vi "Bounded Confidence interval.vi"(1 "Analysis_info_cluster":T1={"Colour"=0, "Inst type"=enum."Pitot-static tube", "Inst name"="Manometer voltage", "Symbol"="U", "Code name"="", "Extra Info"="U", "Inst Array"=enum."PWA", "U"=0.0, "u^2"=0.0, "u^3"=0.0, "u^4"=0.0, "Skew_u"=0.0, "Kurt_u"=0.0, "Sd Error in Mean"=0.0, "% u'/U"=0.0, "X"=0.0, "Y"=0.0, "Z"=0.0, "Timescale integral Estimate"=0.0, "Sd Error in Variance"=0.0, "Calib File"=path "", "Calib Constants"=[], "Output Position"=FALSE, "Stats"=enum."None", "Av Sampling Rate"=0.0, "Av No of Samples"=0.0, "Total Meas Time (s)"=0.0, "OrigChName"="", "Max value"=0.0, "Min value"=0.0, "Req Sample Rate Hz"=0.0, "Sync Delay Time (s)"=0.0, "Ch No"=0, "Device"="", "Use Latest Calib"=FALSE, "Port"="", "Metadata Ch Names"=[], "Metadata Ch Values"=[], "Label"="", "chState"=enum."Solo", "Point Drift"=0.0, "inputConfig"=""} {"Kurt_u" format="%_3g"; "u^4" format="%_3g"; "u^3" format="%_3g"; "Sd Error in Variance" format="%_3g"; "u^2" format="%_3g"; "Sd Error in Mean" format="%_3g"; "U" format="%_3g"; "Sync Delay Time (s)" format="%.4f"; "Total Meas Time (s)" format="%_5g"; "Skew_u" format="%_3g"; "% u'/U" format="%_3g"}, 2 "Lower limit scale factor on SD or SE":dbl, 3 "Upper limit scale factor on SD or SE":dbl) -> (0 "Error values":string[](array[string]))   [LabVIEW 2022 SP3]
uses:
  Controls/Inst_type.ctl
  Controls/Instrument_Array.ctl
  Controls/Analysis_info_cluster.ctl
  Controls/channelState.ctl
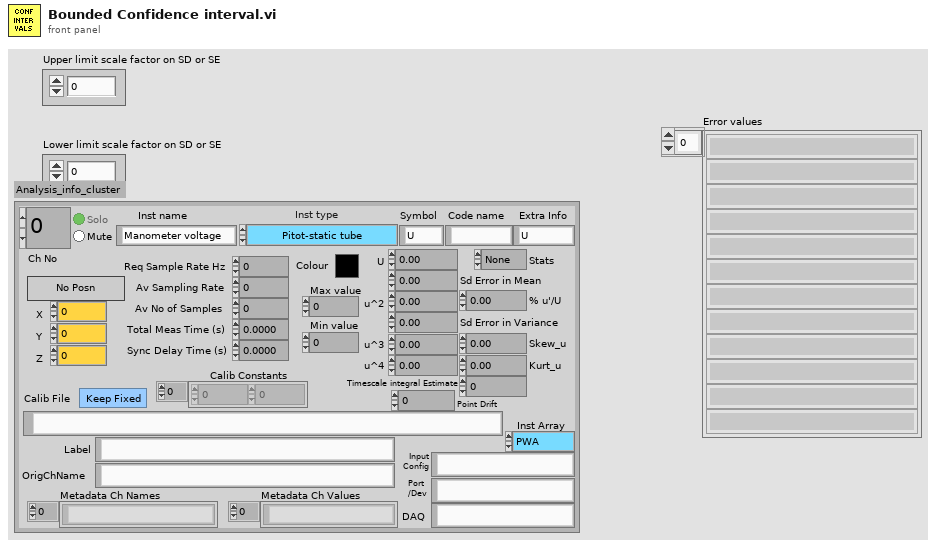
[diagram p1: front panel]
types:
  T1 = typedef "Analysis_info_cluster.ctl" = cluster{"Colour":u32, "Inst type":T2, "Inst name":string, "Symbol":string, "Code name":string, "Extra Info":string, "Inst Array":T3, "U":dbl, "u^2":dbl, "u^3":dbl, "u^4":dbl, "Skew_u":dbl, "Kurt_u":dbl, "Sd Error in Mean":dbl, "% u'/U":dbl, "X":dbl, "Y":dbl, "Z":dbl, "Timescale integral Estimate":dbl, "Sd Error in Variance":dbl, "Calib File":path, "Calib Constants":dbl[], "Output Position":bool, "Stats":enum16{"None", "Basic", "Full"}, "Av Sampling Rate":dbl, "Av No of Samples":dbl, "Total Meas Time (s)":dbl, "OrigChName":string, "Max value":dbl, "Min value":dbl, "Req Sample Rate Hz":dbl, "Sync Delay Time (s)":dbl, "Ch No":i16, "Device":string, "Use Latest Calib":bool, "Port":string, "Metadata Ch Names":string[], "Metadata Ch Values":string[], "Label":string, "chState":T4, "Point Drift":dbl, "inputConfig":string}
  T2 = typedef "Inst_type.ctl" = enum16{"Raw voltage", "Raw with zero offsetting", "Propeller anemometer", "Pressure Transducer", "Pitot-static tube", "Hot wire", "Cross wire 1", "Cross wire 2", "Generic Linear", "Generic Polynomial", "Generic BackPoly", "Fast FID", "Thermocouple", "Cold wire", "Pulsed Wire", "LDA Vel", "LDA Tran time", "LDA Arr time", "Microphone"}
  T3 = typedef "Instrument_Array.ctl" = enum16{"PWA", "LDA", "Analogue"}
  T4 = typedef "channelState.ctl" = enum32{"No Selection", "Solo", "Mute"}
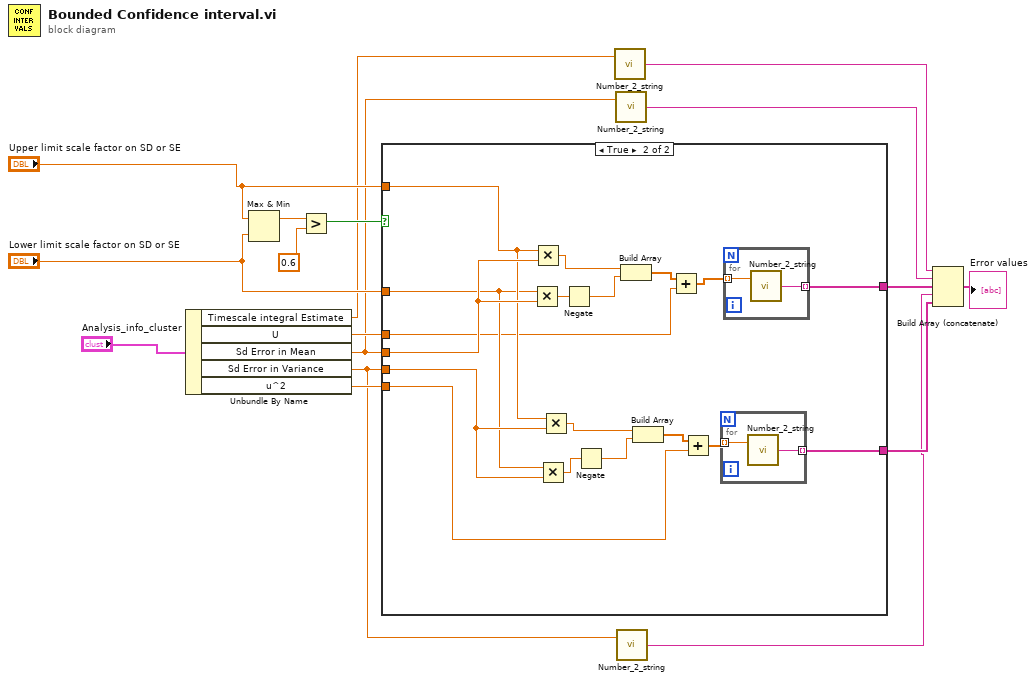
[diagram p0: block diagram]
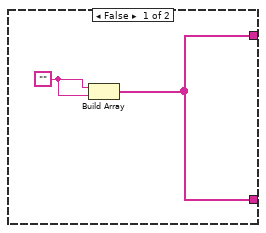
[diagram p2: hidden frame]
diagram:
  n1 = Unbundle By Name("Analysis_info_cluster") -> ("Timescale integral Estimate"=w2:dbl, "U"=w11:dbl, "Sd Error in Mean"=w8:dbl, "Sd Error in Variance"=w5:dbl, "u^2"=w10:dbl)
  n2 = Max & Min(x="Upper limit scale factor on SD or SE", y="Lower limit scale factor on SD or SE") -> (max(x,y)=w16:dbl)  [unwired: 1 out]
  n3 = Greater?(x=w16, y=0.6) -> (0:w14:bool)
  n4 = case shown="True" w14 {
    tunnel: w8 -> [_ w37]
    tunnel: "Upper limit scale factor on SD or SE" -> [_ w36]
    tunnel: "Lower limit scale factor on SD or SE" -> [_ w34]
    tunnel: w5 -> [_ w35]
    tunnel: w11 -> [_ w30]
    tunnel: w10 -> [_ w24]
    tunnel: [w18 w21] -> w9
    tunnel: [w18 w20] -> w6
    frame False {
      w19 = ""
      n5 = Build Array(w19, w19) -> (w18:string[])
    }
    frame True {
      n6 = Multiply(x=w34, y=w37) -> (x*y=w32:dbl)
      n7 = Multiply(x=w36, y=w37) -> (x*y=w33:dbl)
      n8 = Multiply(x=w34, y=w35) -> (x*y=w25:dbl)
      n9 = Multiply(x=w36, y=w35) -> (x*y=w26:dbl)
      n10 = Negate(x=w32) -> (-x=w29:dbl)
      n11 = Negate(x=w25) -> (-x=w28:dbl)
      n12 = Build Array(w33, w29) -> (w31:dbl[])
      n13 = Build Array(w26, w28) -> (w27:dbl[])
      n14 = Add(x=w31, y=w30) -> (x+y=w23:dbl[])
      n15 = Add(x=w27, y=w24) -> (x+y=w22:dbl[])
      n16 = for {
        tunnel: w22 -> [w39] mode=indexing
        tunnel: [w38] -> w20 mode=indexing
        n17 = call "Number_2_string.vi"("number"=w39) -> ("String"=w38:string)  [unwired: 1 in]
      }
      n18 = for {
        tunnel: w23 -> [w41] mode=indexing
        tunnel: [w40] -> w21 mode=indexing
        n19 = call "Number_2_string.vi"("number"=w41) -> ("String"=w40:string)  [unwired: 1 in]
      }
    }
  }
  n20 = call "Number_2_string.vi"("number"=w2) -> ("String"=w1:string)  [unwired: 1 in]
  n21 = call "Number_2_string.vi"("number"=w8) -> ("String"=w7:string)  [unwired: 1 in]
  n22 = call "Number_2_string.vi"("number"=w5) -> ("String"=w4:string)  [unwired: 1 in]
  n23 = Build Array (concatenate)(w1, w7, w9, w4, w6) -> (→"Error values":string[])
